vi "data to bytestream.vi"(7 "big endian?":bool, 9 "specifications":T1[](array[typedef]), 10 "byte allocation":u8[](array[numeric]), 11 "data table":T3) -> (2 "bytestream":u8[](array[numeric]), 3 "allocation":T3)   [LabVIEW 2013, in "EthernetIP runtime.lvclass"]
uses:
  EthernetIP runtime.lvclass
  <vilib>/NI/Tag Bus/table/data table.ctl
  conversion specification.ctl
  <vilib>/NI/Tag Bus/tag/Data Type.ctl
  <vilib>/NI/Tag Bus/table/data polymorphs/read one/read Double.vi
  <vilib>/NI/Tag Bus/table/data polymorphs/read one/read Single.vi
  <vilib>/NI/Tag Bus/table/data polymorphs/read one/read I64.vi
  <vilib>/NI/Tag Bus/table/data polymorphs/read one/read U64.vi
  <vilib>/NI/Tag Bus/table/data polymorphs/read one/read I32.vi
  <vilib>/NI/Tag Bus/table/data polymorphs/read one/read U32.vi
  <vilib>/NI/Tag Bus/table/data polymorphs/read one/read I16.vi
  <vilib>/NI/Tag Bus/table/data polymorphs/read one/read U16.vi
  <vilib>/NI/Tag Bus/table/data polymorphs/read one/read I8.vi
  <vilib>/NI/Tag Bus/table/data polymorphs/read one/read U8.vi
  <vilib>/NI/Tag Bus/table/data polymorphs/read one/read Boolean.vi
  <vilib>/NI/Tag Bus/table/data polymorphs/read one/read Array of Double.vi
  <vilib>/NI/Tag Bus/table/data polymorphs/read one/read Array of Single.vi
  <vilib>/NI/Tag Bus/table/data polymorphs/read one/read Array of I64.vi
  <vilib>/NI/Tag Bus/table/data polymorphs/read one/read Array of I32.vi
  <vilib>/NI/Tag Bus/table/data polymorphs/read one/read Array of I16.vi
  <vilib>/NI/Tag Bus/table/data polymorphs/read one/read Array of I8.vi
  <vilib>/NI/Tag Bus/table/data polymorphs/read one/read Array of U64.vi
  <vilib>/NI/Tag Bus/table/data polymorphs/read one/read Array of U32.vi
  <vilib>/NI/Tag Bus/table/data polymorphs/read one/read Array of U16.vi
  <vilib>/NI/Tag Bus/table/data polymorphs/read one/read Array of U8.vi
  <vilib>/NI/Tag Bus/table/data table.lvlib
  <vilib>/NI/Tag Bus/tag/tag descriptor.lvclass
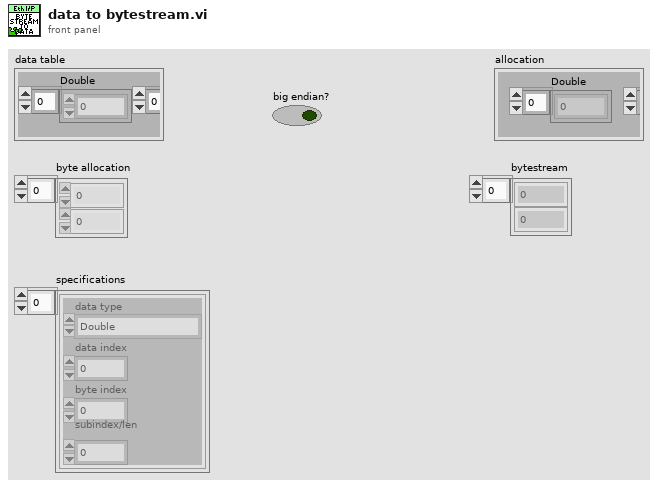
[diagram p1: front panel]
types:
  T1 = typedef "EthernetIP runtime.lvclass/conversion specification.ctl" = cluster{"data type":T2, "data index":i32, "byte index":i32, "subindex/len":i32}
  T2 = typedef "tag bus.lvlib/tag descriptor.lvclass/Data Type.ctl" = enum16{"Double", "Single", "I64", "I32", "I16", "I8", "U64", "U32", "U16", "U8", "Boolean", "String", "Array of Double", "Array of Single", "Array of I64", "Array of I32", "Array of I16", "Array of I8", "Array of U64", "Array of U32", "Array of U16", "Array of U8", "Array of Boolean", "Array of String"}
  T3 = typedef "tag bus.lvlib/data table.lvlib/data table.ctl" = cluster{"Double":dbl[], "Single":sgl[], "I64":i64[], "I32":i32[], "I16":i16[], "I8":i8[], "U64":u64[], "U32":u32[], "U16":u16[], "U8":u8[], "Boolean":bool[], "String":string[], "Array of Double":cluster{"DBL Array":dbl[]}[], "Array of Single":cluster{"SGL Array":sgl[]}[], "Array of I64":cluster{"I64 Array":i64[]}[], "Array of I32":cluster{"I32 Array":i32[]}[], "Array of I16":cluster{"I16 Array":i16[]}[], "Array of I8":cluster{"I8 Array":i8[]}[], "Array of U64":cluster{"U64 Array":u64[]}[], "Array of U32":cluster{"U32 Array":u32[]}[], "Array of U16":cluster{"U16 Array":u16[]}[], "Array of U8":cluster{"U8 Array":u8[]}[], "Array of Boolean":cluster{"Boolean Array":bool[]}[], "Array of String":cluster{"String Array":string[]}[]}
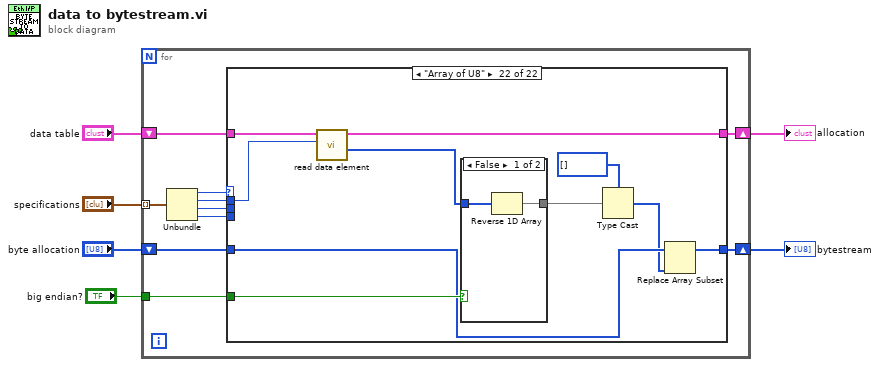
[diagram p0: block diagram]
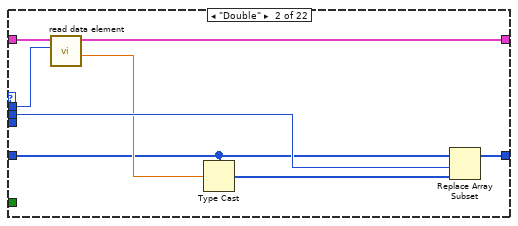
[diagram p3: hidden frame]
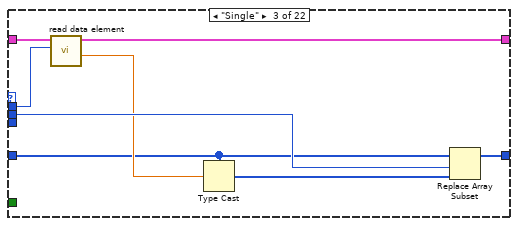
[diagram p4: hidden frame]
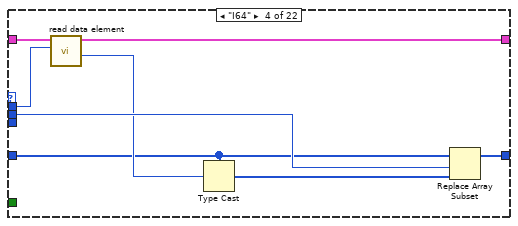
[diagram p5: hidden frame]
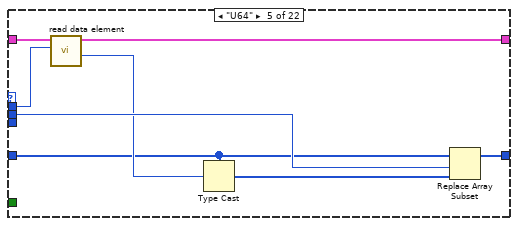
[diagram p6: hidden frame]
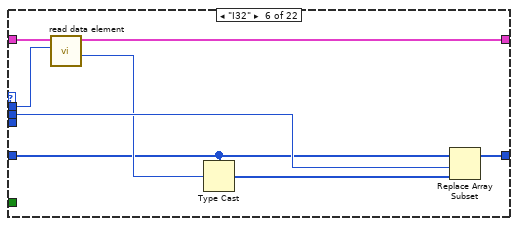
[diagram p7: hidden frame]
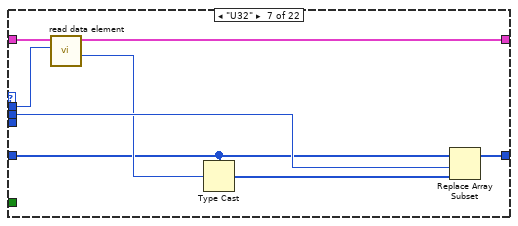
[diagram p8: hidden frame]
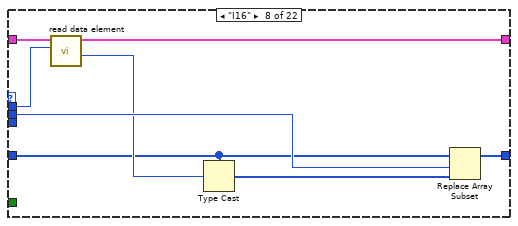
[diagram p9: hidden frame]
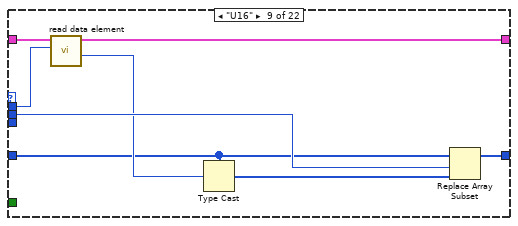
[diagram p10: hidden frame]
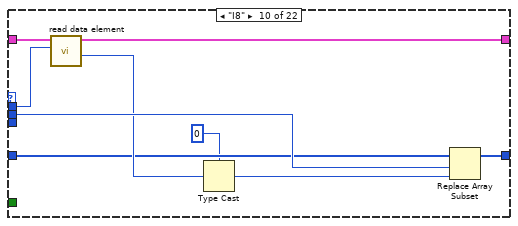
[diagram p11: hidden frame]
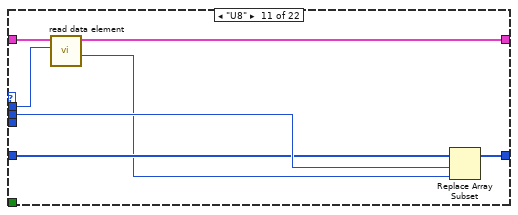
[diagram p12: hidden frame]
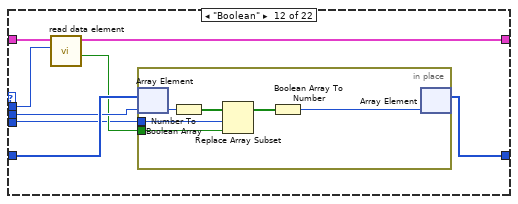
[diagram p13: hidden frame]
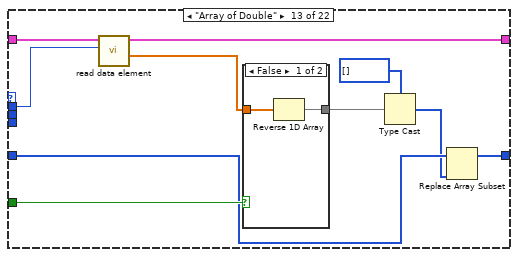
[diagram p14: hidden frame]
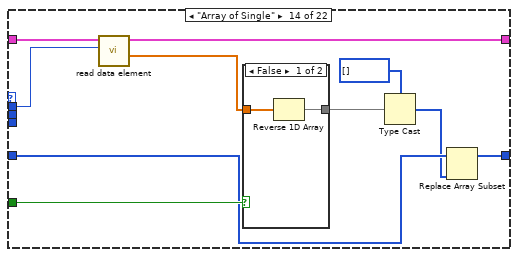
[diagram p16: hidden frame]
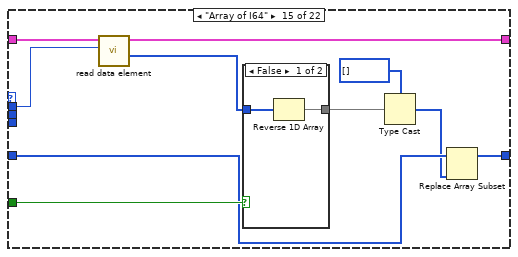
[diagram p18: hidden frame]
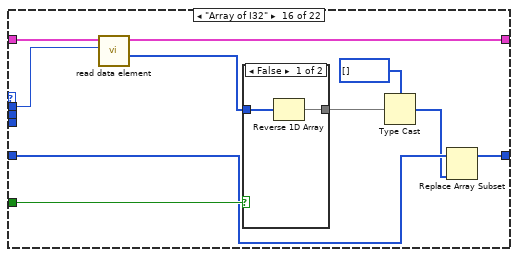
[diagram p20: hidden frame]
diagram:
  n1 = for {
    shift-right: [w13] -> w5
    shift-left: "data table" -> [w14]
    tunnel: "specifications" -> [w16] mode=indexing
    shift-right: [w9] -> w2
    shift-left: "byte allocation" -> [w12]
    tunnel: "big endian?" -> [w7]
    n2 = Unbundle(w16) -> ("data type"=w15:T2, "data index"=w11:i32, "byte index"=w8:i32, "subindex/len"=w10:i32)
    n3 = case shown="\"Array of U8\"" w15 {
      tunnel: w14 -> [w18 w26 w34 w42 w50 w58 w66 w74 w82 w91 w98 w106 w122 w135 w148 w161 w174 w187 w200 w213 w226 w239]
      tunnel: [w18 w25 w33 w41 w49 w57 w65 w73 w81 w90 w97 w105 w121 w134 w147 w160 w173 w186 w199 w212 w225 w238] -> w13
      tunnel: w8 -> [_ w22 w30 w38 w46 w54 w62 w70 w78 w87 w94 w101 _ _ _ _ _ _ _ _ _ _]
      tunnel: w12 -> [w17 w20 w28 w36 w44 w52 w60 w68 w76 w85 w93 w103 w115 w128 w141 w154 w167 w180 w193 w206 w219 w232]
      tunnel: w11 -> [_ w24 w32 w40 w48 w56 w64 w72 w80 w89 w96 w104 w120 w133 w146 w159 w172 w185 w198 w211 w224 w237]
      tunnel: w10 -> [_ _ _ _ _ _ _ _ _ _ _ w99 _ _ _ _ _ _ _ _ _ _]
      tunnel: [w17 w23 w31 w39 w47 w55 w63 w71 w79 w88 w95 w102 w114 w127 w140 w153 w166 w179 w192 w205 w218 w231] -> w9
      tunnel: w7 -> [_ _ _ _ _ _ _ _ _ _ _ _ w119 w132 w145 w158 w171 w184 w197 w210 w223 w236]
      frame Default {
      }
      frame "Double" {
        n4 = call-poly <vilib>:"read data element.vi"("index"=w24, "data table in"=w26) -> ("value"=w21:dbl, "data table out"=w25:T3)  [unwired: 8 in]
        n5 = Type Cast(type=w20, x=w21) -> (*(type *) &x=w19:u8[])
        n6 = Replace Array Subset(array=w20, new element=w19, index=w22) -> (w23:u8[])
      }
      frame "Single" {
        n7 = call-poly <vilib>:"read data element.vi"("index"=w32, "data table in"=w34) -> ("value"=w29:sgl, "data table out"=w33:T3)  [unwired: 8 in]
        n8 = Type Cast(type=w28, x=w29) -> (*(type *) &x=w27:u8[])
        n9 = Replace Array Subset(array=w28, new element=w27, index=w30) -> (w31:u8[])
      }
      frame "I64" {
        n10 = call-poly <vilib>:"read data element.vi"("index"=w40, "data table in"=w42) -> ("value"=w37:i64, "data table out"=w41:T3)  [unwired: 8 in]
        n11 = Type Cast(type=w36, x=w37) -> (*(type *) &x=w35:u8[])
        n12 = Replace Array Subset(array=w36, new element=w35, index=w38) -> (w39:u8[])
      }
      frame "U64" {
        n13 = call-poly <vilib>:"read data element.vi"("index"=w48, "data table in"=w50) -> ("value"=w45:u64, "data table out"=w49:T3)  [unwired: 8 in]
        n14 = Type Cast(type=w44, x=w45) -> (*(type *) &x=w43:u8[])
        n15 = Replace Array Subset(array=w44, new element=w43, index=w46) -> (w47:u8[])
      }
      frame "I32" {
        n16 = call-poly <vilib>:"read data element.vi"("index"=w56, "data table in"=w58) -> ("value"=w53:i32, "data table out"=w57:T3)  [unwired: 8 in]
        n17 = Type Cast(type=w52, x=w53) -> (*(type *) &x=w51:u8[])
        n18 = Replace Array Subset(array=w52, new element=w51, index=w54) -> (w55:u8[])
      }
      frame "U32" {
        n19 = call-poly <vilib>:"read data element.vi"("index"=w64, "data table in"=w66) -> ("value"=w61:u32, "data table out"=w65:T3)  [unwired: 8 in]
        n20 = Type Cast(type=w60, x=w61) -> (*(type *) &x=w59:u8[])
        n21 = Replace Array Subset(array=w60, new element=w59, index=w62) -> (w63:u8[])
      }
      frame "I16" {
        n22 = call-poly <vilib>:"read data element.vi"("index"=w72, "data table in"=w74) -> ("value"=w69:i16, "data table out"=w73:T3)  [unwired: 8 in]
        n23 = Type Cast(type=w68, x=w69) -> (*(type *) &x=w67:u8[])
        n24 = Replace Array Subset(array=w68, new element=w67, index=w70) -> (w71:u8[])
      }
      frame "U16" {
        n25 = call-poly <vilib>:"read data element.vi"("index"=w80, "data table in"=w82) -> ("value"=w77:u16, "data table out"=w81:T3)  [unwired: 8 in]
        n26 = Type Cast(type=w76, x=w77) -> (*(type *) &x=w75:u8[])
        n27 = Replace Array Subset(array=w76, new element=w75, index=w78) -> (w79:u8[])
      }
      frame "I8" {
        n28 = call-poly <vilib>:"read data element.vi"("index"=w89, "data table in"=w91) -> ("value"=w86:i8, "data table out"=w90:T3)  [unwired: 8 in]
        n29 = Type Cast(type=u8 0, x=w86) -> (*(type *) &x=w84:u8)
        n30 = Replace Array Subset(array=w85, new element=w84, index=w87) -> (w88:u8[])
      }
      frame "U8" {
        n31 = call-poly <vilib>:"read data element.vi"("index"=w96, "data table in"=w98) -> ("value"=w92:u8, "data table out"=w97:T3)  [unwired: 8 in]
        n32 = Replace Array Subset(array=w93, new element=w92, index=w94) -> (w95:u8[])
      }
      frame "Boolean" {
        n33 = call-poly <vilib>:"read data element.vi"("index"=w104, "data table in"=w106) -> ("value"=w100:bool, "data table out"=w105:T3)  [unwired: 8 in]
        n34 = in-place {
          in-place-border: w100 -> [w108]
          in-place-border: w99 -> [w107]
          n35 = in-place-array #1(w103, w101) -> (w112:u8)
          n36 = Number To Boolean Array(number=w112) -> (Boolean array=w110:bool[])
          n37 = Replace Array Subset(array=w110, new element=w108, index=w107) -> (w109:bool[])
          n38 = Boolean Array To Number(Boolean array=w109) -> (number=w111:u8)
          n39 = in-place-array #1(w111) -> (w102:u8[])  [unwired: 1 out]
        }
      }
      frame "Array of Double" {
        n40 = call-poly <vilib>:"read data element.vi"("index"=w120, "data table in"=w122) -> ("value"=w118:dbl[], "data table out"=w121:T3)  [unwired: 8 in]
        n41 = case shown="False" w119 {
          tunnel: w118 -> [w124 w125]
          tunnel: [w123 w125] -> w117
          frame False {
            n42 = Reverse 1D Array(array=w124) -> (reversed array=w123:dbl[])
          }
          frame True {
          }
        }
        n43 = Type Cast(type=u8[] [] ("byte allocation"), x=w117) -> (*(type *) &x=w113:u8[])
        n44 = Replace Array Subset(array=w115, new element=w113) -> (w114:u8[])  [unwired: 1 in]
      }
      frame "Array of Single" {
        n45 = call-poly <vilib>:"read data element.vi"("index"=w133, "data table in"=w135) -> ("value"=w131:sgl[], "data table out"=w134:T3)  [unwired: 8 in]
        n46 = case shown="False" w132 {
          tunnel: w131 -> [w137 w138]
          tunnel: [w136 w138] -> w130
          frame False {
            n47 = Reverse 1D Array(array=w137) -> (reversed array=w136:sgl[])
          }
          frame True {
          }
        }
        n48 = Type Cast(type=u8[] [] ("byte allocation"), x=w130) -> (*(type *) &x=w126:u8[])
        n49 = Replace Array Subset(array=w128, new element=w126) -> (w127:u8[])  [unwired: 1 in]
      }
      frame "Array of I64" {
        n50 = call-poly <vilib>:"read data element.vi"("index"=w146, "data table in"=w148) -> ("value"=w144:i64[], "data table out"=w147:T3)  [unwired: 8 in]
        n51 = case shown="False" w145 {
          tunnel: w144 -> [w150 w151]
          tunnel: [w149 w151] -> w143
          frame False {
            n52 = Reverse 1D Array(array=w150) -> (reversed array=w149:i64[])
          }
          frame True {
          }
        }
        n53 = Type Cast(type=u8[] [] ("byte allocation"), x=w143) -> (*(type *) &x=w139:u8[])
        n54 = Replace Array Subset(array=w141, new element=w139) -> (w140:u8[])  [unwired: 1 in]
      }
      frame "Array of I32" {
        n55 = call-poly <vilib>:"read data element.vi"("index"=w159, "data table in"=w161) -> ("value"=w157:i32[], "data table out"=w160:T3)  [unwired: 8 in]
        n56 = case shown="False" w158 {
          tunnel: w157 -> [w163 w164]
          tunnel: [w162 w164] -> w156
          frame False {
            n57 = Reverse 1D Array(array=w163) -> (reversed array=w162:i32[])
          }
          frame True {
          }
        }
        n58 = Type Cast(type=u8[] [] ("byte allocation"), x=w156) -> (*(type *) &x=w152:u8[])
        n59 = Replace Array Subset(array=w154, new element=w152) -> (w153:u8[])  [unwired: 1 in]
      }
      frame "Array of I16" {
        n60 = call-poly <vilib>:"read data element.vi"("index"=w172, "data table in"=w174) -> ("value"=w170:i16[], "data table out"=w173:T3)  [unwired: 8 in]
        n61 = case shown="False" w171 {
          tunnel: w170 -> [w176 w177]
          tunnel: [w175 w177] -> w169
          frame False {
            n62 = Reverse 1D Array(array=w176) -> (reversed array=w175:i16[])
          }
          frame True {
          }
        }
        n63 = Type Cast(type=u8[] [] ("byte allocation"), x=w169) -> (*(type *) &x=w165:u8[])
        n64 = Replace Array Subset(array=w167, new element=w165) -> (w166:u8[])  [unwired: 1 in]
      }
      frame "Array of I8" {
        n65 = call-poly <vilib>:"read data element.vi"("index"=w185, "data table in"=w187) -> ("value"=w183:i8[], "data table out"=w186:T3)  [unwired: 8 in]
        n66 = case shown="False" w184 {
          tunnel: w183 -> [w189 w190]
          tunnel: [w188 w190] -> w182
          frame False {
            n67 = Reverse 1D Array(array=w189) -> (reversed array=w188:i8[])
          }
          frame True {
          }
        }
        n68 = Type Cast(type=u8[] [] ("byte allocation"), x=w182) -> (*(type *) &x=w178:u8[])
        n69 = Replace Array Subset(array=w180, new element=w178) -> (w179:u8[])  [unwired: 1 in]
      }
      frame "Array of U64" {
        n70 = call-poly <vilib>:"read data element.vi"("index"=w198, "data table in"=w200) -> ("value"=w196:u64[], "data table out"=w199:T3)  [unwired: 8 in]
        n71 = case shown="False" w197 {
          tunnel: w196 -> [w202 w203]
          tunnel: [w201 w203] -> w195
          frame False {
            n72 = Reverse 1D Array(array=w202) -> (reversed array=w201:u64[])
          }
          frame True {
          }
        }
        n73 = Type Cast(type=u8[] [] ("byte allocation"), x=w195) -> (*(type *) &x=w191:u8[])
        n74 = Replace Array Subset(array=w193, new element=w191) -> (w192:u8[])  [unwired: 1 in]
      }
      frame "Array of U32" {
        n75 = call-poly <vilib>:"read data element.vi"("index"=w211, "data table in"=w213) -> ("value"=w209:u32[], "data table out"=w212:T3)  [unwired: 8 in]
        n76 = case shown="False" w210 {
          tunnel: w209 -> [w215 w216]
          tunnel: [w214 w216] -> w208
          frame False {
            n77 = Reverse 1D Array(array=w215) -> (reversed array=w214:u32[])
          }
          frame True {
          }
        }
        n78 = Type Cast(type=u8[] [] ("byte allocation"), x=w208) -> (*(type *) &x=w204:u8[])
        n79 = Replace Array Subset(array=w206, new element=w204) -> (w205:u8[])  [unwired: 1 in]
      }
      frame "Array of U16" {
        n80 = call-poly <vilib>:"read data element.vi"("index"=w224, "data table in"=w226) -> ("value"=w222:u16[], "data table out"=w225:T3)  [unwired: 8 in]
        n81 = case shown="False" w223 {
          tunnel: w222 -> [w228 w229]
          tunnel: [w227 w229] -> w221
          frame False {
            n82 = Reverse 1D Array(array=w228) -> (reversed array=w227:u16[])
          }
          frame True {
          }
        }
        n83 = Type Cast(type=u8[] [] ("byte allocation"), x=w221) -> (*(type *) &x=w217:u8[])
        n84 = Replace Array Subset(array=w219, new element=w217) -> (w218:u8[])  [unwired: 1 in]
      }
      frame "Array of U8" {
        n85 = call-poly <vilib>:"read data element.vi"("index"=w237, "data table in"=w239) -> ("value"=w235:u8[], "data table out"=w238:T3)  [unwired: 8 in]
        n86 = case shown="False" w236 {
          tunnel: w235 -> [w241 w242]
          tunnel: [w240 w242] -> w234
          frame False {
            n87 = Reverse 1D Array(array=w241) -> (reversed array=w240:u8[])
          }
          frame True {
          }
        }
        n88 = Type Cast(type=u8[] [] ("byte allocation"), x=w234) -> (*(type *) &x=w230:u8[])
        n89 = Replace Array Subset(array=w232, new element=w230) -> (w231:u8[])  [unwired: 1 in]
      }
    }
  }
  "allocation" <- w5
  "bytestream" <- w2
